vi "destring_notifier_values.vi"(11 "input cluster":cluster{"names":string, "value":variant}) -> (2 "Array 2":string[](array[string]), 3 "Array":string[](array[string]))   [LabVIEW 2013]
doc: "Takes a stringifed notifier and reads out the values"
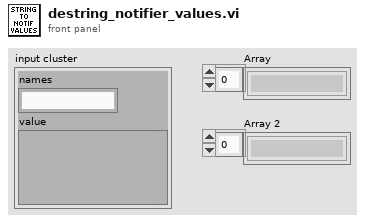
[diagram p1: front panel]
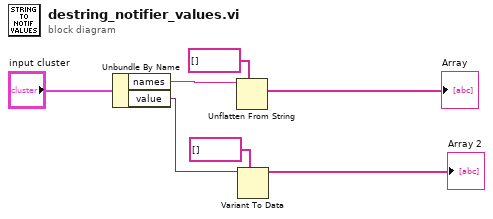
[diagram p0: block diagram]
diagram:
  n1 = Unbundle By Name("input cluster") -> ("names"=w4:string, "value"=w6:variant)
  n2 = Unflatten From String(type=string[] [], binary string=w4) -> (value=→"Array":string[])  [unwired: 3 in, 2 out]
  n3 = Variant To Data(type=string[] [], Variant=w6) -> (data=→"Array 2":string[])  [unwired: 1 in, 1 out]
